vi "Conditions that are TRUE (active rules).vi"(8 "error in (no error)":errorcluster, 10 "Active rules":bool[](array[boolean])) -> (0 "error out":errorcluster)   [LabVIEW 2018, in "TTL IO.lvlib"]
doc: "<b>Note</b>: This VI was renamed by the DQMH Rename Event utility. Make sure the VI Description is updated to reflect the new event name, then delete this comment.\n\nShows which rules are currecntly TRUE.\n_____\nCreated using Delacor QMH Event Scripter 4.2.1.88."
uses:
  TTL IO.lvlib
  Conditions that are TRUE (active rules) Argument--cluster.ctl
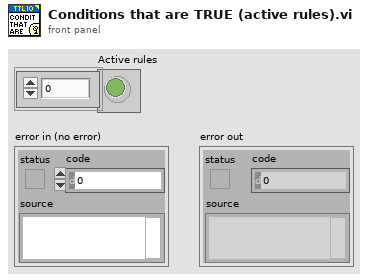
[diagram p1: front panel]
types:
  T1 = typedef "TTL IO.lvlib/Conditions that are TRUE (active rules) Argument--cluster.ctl" = cluster{"Active rules":bool[]}
  T2 = typedef "TTL IO.lvlib/Broadcast Events--cluster.ctl" = cluster{"Module Did Init":refnum<user-event>, "Status Updated":refnum<user-event>, "Error Reported":refnum<user-event>, "Module Did Stop":refnum<user-event>, "Update Module Execution Status":refnum<user-event>, "Conditions that are TRUE (active rules)":refnum<user-event>}
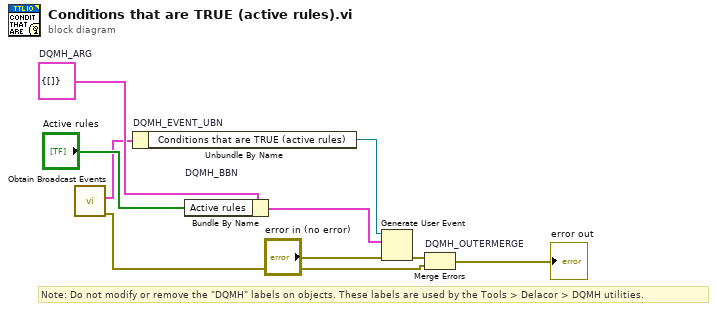
[diagram p0: block diagram]
diagram:
  w4 = T1 {"Active rules"=[]}  # DQMH_ARG
  # "Note: Do not modify or remove the \"DQMH\" labels on objects. These labels are used by the Tools > Delacor > DQMH utilities."
  n1 = call "Obtain Broadcast Events.vi"() -> ("error out"=w2:errorcluster, "TTL IO Broadcast Events"=w1:T2)  [unwired: 10 in]
  n2 = Unbundle By Name "DQMH_EVENT_UBN"(w1) -> ("Conditions that are TRUE (active rules)"=w6:refnum<user-event>)
  n3 = Bundle By Name "DQMH_BBN"(cluster=w4, "Active rules"="Active rules") -> (w7:T1)
  n4 = Generate User Event(user event=w6, event data cluster=w7, error in="error in (no error)") -> (error out=w5:errorcluster)  [unwired: 1 in, 1 out]
  n5 = Merge Errors "DQMH_OUTERMERGE"(w5, w2) -> (→"error out":errorcluster)
